vi "5-k-dist.vi"(0 "Loi de Poisson":T1 caption="p_POI", 5 "k":i32, 11 "error in":errorcluster caption="err in") -> (4 "Loi de Poisson":T1 caption="p_POI", 6 "k":i32, 8 "p(X=k)":dbl, 10 "F(X<=k)":dbl, 15 "error out":errorcluster caption="err out")   [LabVIEW 2010, in "lv_02.lvlib"]
uses:
  p_5E5_LPoi.ctl
  <vilib>/gmath/statdist.llb/Poisson CDF.vi
  <vilib>/gmath/statdist.llb/Poisson PF.vi
  lv_02.lvlib
  <vilib>/gmath/NI_Gmath.lvlib
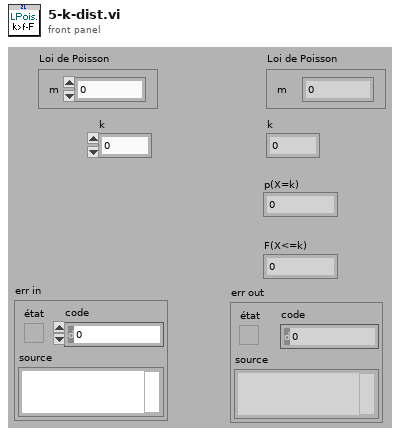
[diagram p1: front panel]
types:
  T1 = typedef "lv_02.lvlib/p_5E5_LPoi.ctl" = cluster{"m":dbl}
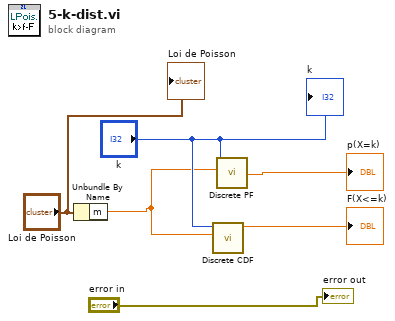
[diagram p0: block diagram]
diagram:
  n1 = Unbundle By Name("Loi de Poisson") -> ("m"=w1:dbl)
  n2 = call-poly <vilib>:"Discrete CDF.vi"("lambda"=w1, "x"="k") -> ("cdf(x)"=→"F(X<=k)":dbl)  [unwired: 8 in, 1 out]
  n3 = call-poly <vilib>:"Discrete PF.vi"("lambda"=w1, "x"="k") -> ("prob(x)"=→"p(X=k)":dbl)  [unwired: 8 in, 1 out]
  "error out" <- "error in"
  "Loi de Poisson" <- "Loi de Poisson"
  "k" <- "k"
